vi "5RobotsPosition.vi"(8 "error in (no error)":errorcluster, 9 "Game":refnum<class "Game.lvclass">, 11 "Utilities in":refnum<class "Utilities.lvclass">) -> (0 "error out":errorcluster, 2 "5Positions":dbl[][](array[numeric]), 3 "Utilities out":refnum<class "Utilities.lvclass">)   [LabVIEW 2023, in "Utilities.lvclass"]
uses:
  Utilities.lvclass
  Game_class/Game.lvclass
  Game_class/Game.lvclass/Game.ctl
  PositionToReceivePassSkill_class/PositionToReceivePassSkill.lvclass
  Robot_class/Robot.lvclass
  Referee_class/command_interpreted.ctl
  Referee_class/Referee.lvclass/Referee.ctl
  Team_class/Read OffensivePlay.vi
  Referee_class/Read command_interpreted.vi
  Game_class/Read BallRef.vi
  Game_class/Read FieldRef.vi
  Game_class/Read Referee.vi
  Game_class/Read AllyRef.vi
  Ball_class/Ball.lvclass
  Field_class/Field.lvclass
  Referee_class/Referee.lvclass
  Ally_class/Ally.lvclass
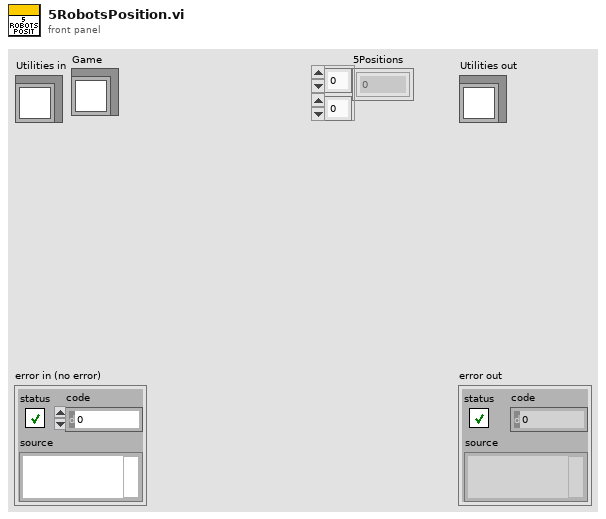
[diagram p1: front panel]
types:
  T1 = typedef "command_interpreted.ctl" = enum16{"Goal Ally", "Goal Enemy", "Ball Placement Enemy", "Ball Placement Ally", "Normal Half Time", "Extra Time  Break", "Extra Half Time", "None", "Post Game", "PKA Normal Start", "Prepare Kickoff Ally", "PKE Normal Start", "Prepare Kickoff Enemy", "Force Start", "Halt", "Timeout", "Prepare Penalty Ally", "Prepare Penalty Enemy", "PPA NormalStart", "PPE Normal Start", "Indirect Free Ally", "Direct Free Enemy", "Direct Free Ally", "Indirect Free Enemy", "Stop"}
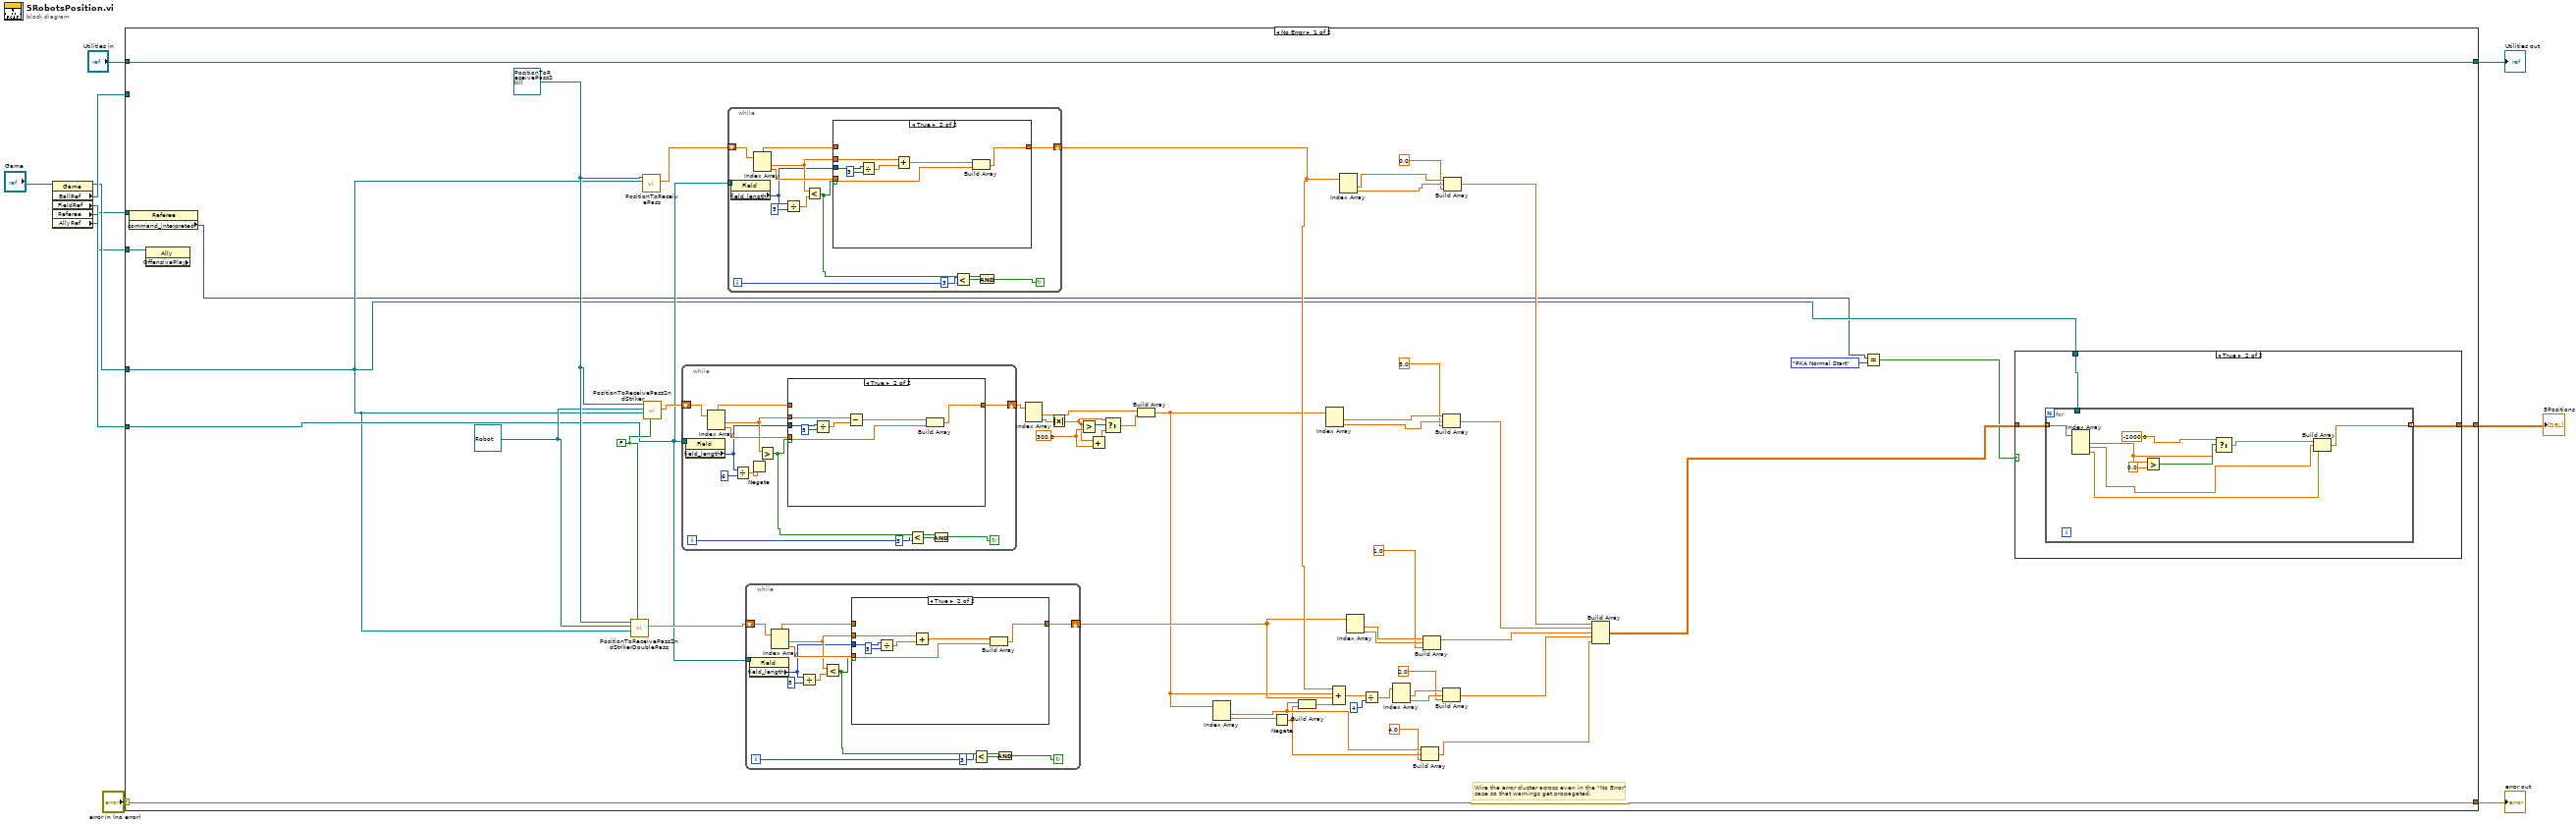
[diagram p0: block diagram]
diagram:
  n1 = property class="Game"(reference="Game") -> (reference out=w4:refnum<class "Game.lvclass">, "BallRef"=w5:refnum<class "Ball.lvclass">, "FieldRef"=w3:refnum<class "Field.lvclass">, "Referee"=w2:refnum<class "Referee.lvclass">, "AllyRef"=w1:refnum<class "Ally.lvclass">)  [unwired: 1 in, 1 out]
  n2 = case shown="No Error" "error in (no error)" {
    selector: "error in (no error)" -> [w64 w143]
    tunnel: [w64 w143] -> w10
    tunnel: [w40 w142] -> w8
    tunnel: "Utilities in" -> [w40 w142]
    tunnel: [w33 _] -> w7
    tunnel: w5 -> [_ _]
    tunnel: w4 -> [w31 _]
    tunnel: w3 -> [w34 _]
    tunnel: w2 -> [w32 _]
    tunnel: w1 -> [w15 _]
    frame No Error {
      w25 = 300.0 ("y")
      w51 = refnum<class "Robot.lvclass"> refnum ("Robot")
      w50 = FALSE ("Boolean")
      w52 = refnum<class "PositionToReceivePassSkill.lvclass"> refnum ("PositionToReceivePassSkill in")
      # "Wire the error cluster across even in the \"No Error\"\ncase so that warnings get propagated."
      n3 = property class="Referee"(reference=w32) -> ("command_interpreted"=w14:T1)  [unwired: 1 in, 2 out]
      n4 = property class="Ally" props=["OffensivePlay"](reference=w15) -> ()  [unwired: 1 in, 3 out]
      n5 = call "PositionToReceivePass2ndStrikerDoublePass.vi"("Boolean"=w50, "Game"=w31, "Robot"=w51, "PositionToReceivePassSkill in"=w52) -> ("2ndStrikerPositionDoublePass"=w35:dbl[])  [unwired: 5 in, 2 out]
      n6 = call-dynamic "PositionToReceivePass.vi"("Game"=w31, "PositionToReceivePassSkill in"=w52) -> ("Position"=w37:dbl[])  [unwired: 7 in, 2 out]
      n7 = call "PositionToReceivePass2ndStriker.vi"("Boolean"=w50, "Game in"=w31, "Robot"=w51, "PositionToReceivePassSkill in"=w52) -> ("2nd Striker Position"=w39:dbl[])  [unwired: 5 in, 2 out]
      n8 = while {
        tunnel: w34 -> [w131]
        shift-right: [w133] -> w30
        shift-left: w39 -> [w132]
        i -> [w126]
        stop <- w127 continue-if-true
        n9 = property class="Field"(reference=w131) -> ("field_length"=w122:i32)  [unwired: 1 in, 2 out]
        n10 = Index Array(array=w132) -> (element #1=w130:dbl, element #2=w129:dbl)  [unwired: 2 in]
        n11 = Divide(x=w122, y=6) -> (x/y=w120:dbl)
        n12 = Negate(x=w120) -> (-x=w121:dbl)
        n13 = Greater?(x=w130, y=w121) -> (0:w128:bool)
        n14 = case shown="True" w128 {
          tunnel: [w134 w141] -> w133
          tunnel: w132 -> [w134 _]
          tunnel: w130 -> [_ w140]
          tunnel: w122 -> [_ w139]
          tunnel: w129 -> [_ w135]
          frame False {
          }
          frame True {
            n15 = Divide(x=w139, y=5) -> (x/y=w137:dbl)
            n16 = Subtract(x=w140, y=w137) -> (x-y=w136:dbl)
            n17 = Build Array(w136, w135) -> (w141:dbl[])
          }
        }
        n18 = Less?(x=w126, y=3) -> (x < y?=w124:bool)
        n19 = And(x=w128, y=w124) -> (x .and. y?=w127:bool)
      }
      n20 = while {
        tunnel: w34 -> [w109]
        shift-right: [w111] -> w38
        shift-left: w37 -> [w110]
        i -> [w106]
        stop <- w107 continue-if-true
        n21 = property class="Field"(reference=w109) -> ("field_length"=w101:i32)  [unwired: 1 in, 2 out]
        n22 = Index Array(array=w110) -> (element #1=w103:dbl, element #2=w108:dbl)  [unwired: 2 in]
        n23 = Divide(x=w101, y=5) -> (x/y=w99:dbl)
        n24 = Less?(x=w103, y=w99) -> (x < y?=w102:bool)
        n25 = case shown="True" w102 {
          tunnel: [w112 w119] -> w111
          tunnel: w110 -> [w112 _]
          tunnel: w103 -> [_ w113]
          tunnel: w101 -> [_ w118]
          tunnel: w108 -> [_ w116]
          frame False {
          }
          frame True {
            n26 = Divide(x=w118, y=5) -> (x/y=w115:dbl)
            n27 = Add(x=w113, y=w115) -> (x+y=w114:dbl)
            n28 = Build Array(w114, w116) -> (w119:dbl[])
          }
        }
        n29 = Less?(x=w106, y=3) -> (x < y?=w104:bool)
        n30 = And(x=w102, y=w104) -> (x .and. y?=w107:bool)
      }
      n31 = while {
        shift-right: [w90] -> w36
        shift-left: w35 -> [w89]
        tunnel: w34 -> [w81]
        i -> [w86]
        stop <- w87 continue-if-true
        n32 = property class="Field"(reference=w81) -> ("field_length"=w79:i32)  [unwired: 1 in, 2 out]
        n33 = Index Array(array=w89) -> (element #1=w83:dbl, element #2=w88:dbl)  [unwired: 2 in]
        n34 = Divide(x=w79, y=5) -> (x/y=w78:dbl)
        n35 = Less?(x=w83, y=w78) -> (x < y?=w82:bool)
        n36 = case shown="True" w82 {
          tunnel: [w91 w98] -> w90
          tunnel: w89 -> [w91 _]
          tunnel: w83 -> [_ w92]
          tunnel: w79 -> [_ w97]
          tunnel: w88 -> [_ w95]
          frame False {
          }
          frame True {
            n37 = Divide(x=w97, y=5) -> (x/y=w94:dbl)
            n38 = Add(x=w92, y=w94) -> (x+y=w93:dbl)
            n39 = Build Array(w93, w95) -> (w98:dbl[])
          }
        }
        n40 = Less?(x=w86, y=3) -> (x < y?=w84:bool)
        n41 = And(x=w82, y=w84) -> (x .and. y?=w87:bool)
      }
      n42 = Index Array(array=w30) -> (element #1=w28:dbl, element #2=w23:dbl)  [unwired: 2 in]
      n43 = Absolute Value(x=w23) -> (abs(x)=w22:dbl)
      n44 = Greater?(x=w22, y=w25) -> (0:w27:bool)
      n45 = Add(x=w22, y=w25) -> (x+y=w24:dbl)
      n46 = Select(t=w22, s=w27, f=w24) -> (s? t:f=w26:dbl)
      n47 = Build Array(w28, w26) -> (w29:dbl[])
      n48 = Index Array(array=w29) -> (element #1=w43:dbl, element #2=w44:dbl)  [unwired: 2 in]
      n49 = Negate(x=w44) -> (-x=w42:dbl)
      n50 = Build Array(w43, w42) -> (w41:dbl[])
      n51 = Index Array(array=w29) -> (element #1=w56:dbl, element #2=w55:dbl)  [unwired: 2 in]
      n52 = Compound Arithmetic op=ADD(w38, w29, w36, w41) -> (w49:dbl[])
      n53 = Index Array(array=w38) -> (element #1=w58:dbl, element #2=w57:dbl)  [unwired: 2 in]
      n54 = Index Array(array=w36) -> (element #1=w54:dbl, element #2=w53:dbl)  [unwired: 2 in]
      n55 = Divide(x=w49, y=4) -> (x/y=w47:dbl[])
      n56 = Index Array(array=w47) -> (element #1=w46:dbl, element #2=w45:dbl)  [unwired: 2 in]
      n57 = Build Array(w43, w42, 4.0) -> (w60:dbl[])
      n58 = Build Array(w54, w53, 1.0) -> (w59:dbl[])
      n59 = Build Array(w56, w55, 3.0) -> (w62:dbl[])
      n60 = Build Array(w46, w45, 2.0) -> (w61:dbl[])
      n61 = Build Array(w58, w57, 0.0) -> (w63:dbl[])
      n62 = Build Array(w63, w62, w59, w61, w60) -> (w21:dbl[][])
      n63 = Equal?(x=w14, y=command_interpreted."PKA Normal Start") -> (x = y?=w12:bool)
      n64 = case shown="True" w12 {
        tunnel: [w65 w66] -> w33
        tunnel: w21 -> [w65 w68]
        tunnel: w31 -> [_ w67]
        frame False {
        }
        frame True {
          n65 = for {
            tunnel: w68 -> [w77] mode=indexing
            tunnel: [w76] -> w66 mode=indexing
            tunnel: w67 -> [_]
            n66 = Index Array(array=w77) -> (element #1=w72:dbl, element #2=w70:dbl, element #3=w69:dbl)  [unwired: 3 in]
            n67 = Greater?(x=w72, y=0.0) -> (0:w74:bool)
            n68 = Select(t=-1000.0 ("x"), s=w74, f=w72) -> (s? t:f=w73:dbl)
            n69 = Build Array(w73, w70, w69) -> (w76:dbl[])
          }
        }
      }
    }
    frame Error {
    }
  }
  "error out" <- w10
  "Utilities out" <- w8
  "5Positions" <- w7
